vi "WriteProtect.vi"(8 "Error In":errorcluster, 10 "Port":bool[](array[boolean]), 11 "Keithley 2602 In":refnum<visa-resource-name>) -> (0 "Error Out":errorcluster, 3 "Keithley 2602 Out":refnum<visa-resource-name>)   [LabVIEW 2012, in "Keithley-2602.lvlib"]
uses:
  Keithley-2602.lvlib
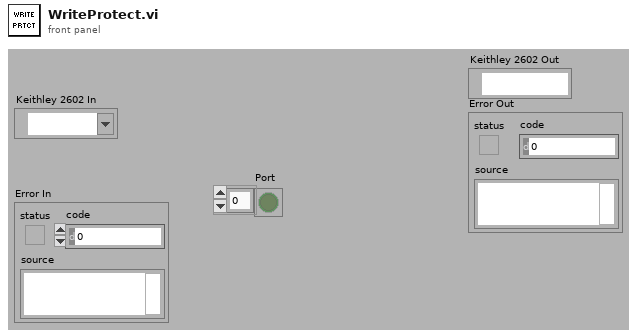
[diagram p1: front panel]
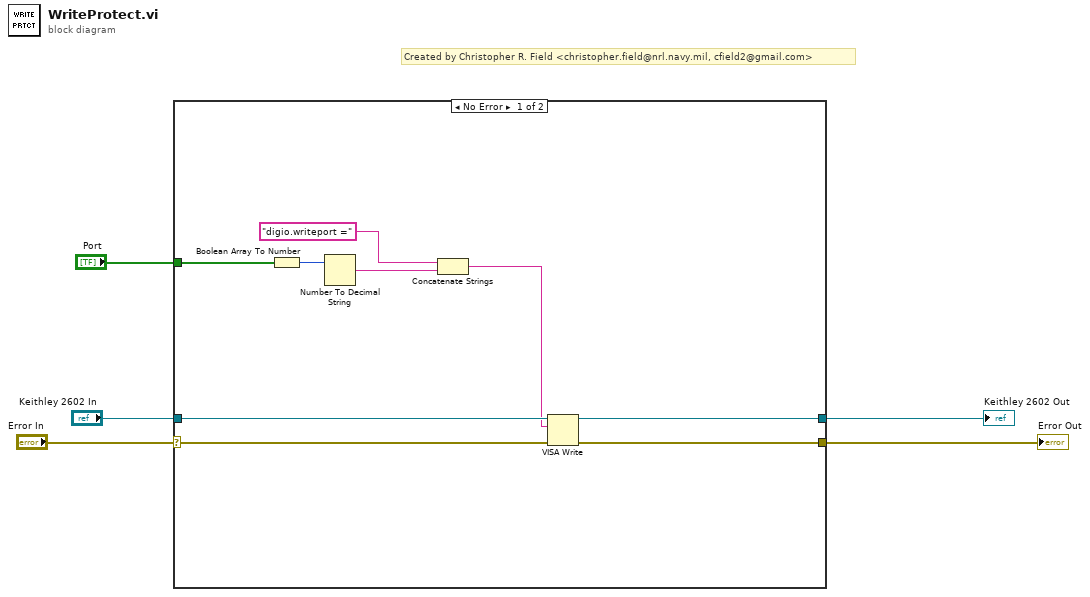
[diagram p0: block diagram]
diagram:
  # "Created by Christopher R. Field <christopher.field@nrl.navy.mil, cfield2@gmail.com>"
  n1 = case shown="No Error" "Error In" {
    selector: "Error In" -> [w6 w15]
    tunnel: "Keithley 2602 In" -> [w14 w16]
    tunnel: [w13 w16] -> w4
    tunnel: [w12 w15] -> w3
    tunnel: "Port" -> [w9 _]
    frame No Error {
      n2 = Boolean Array To Number(Boolean array=w9) -> (number=w8:u32)
      n3 = Number To Decimal String(number=w8) -> (decimal integer string=w7:string)  [unwired: 1 in]
      n4 = Concatenate Strings("digio.writeport =", w7) -> (w10:string)
      n5 = VISA Write(VISA resource name=w14, write buffer=w10, error in (no error)=w6) -> (VISA resource name out=w13:refnum<visa-resource-name>, error out=w12:errorcluster)  [unwired: 1 out]
    }
    frame Error {
    }
  }
  "Keithley 2602 Out" <- w4
  "Error Out" <- w3
